vi "Auton Unbundle Array.vi"(10 "index (col)":i32, 11 "array":dbl[][](array[numeric])) -> (0 "Left Drive":dbl, 1 "Right Drive":dbl, 2 "Right Encoder":dbl, 3 "Auton Left Arm":dbl, 4 "Left Encoder":dbl, 5 "Auton Right Arm":dbl, 6 "Gripper":dbl)   [LabVIEW 2014]
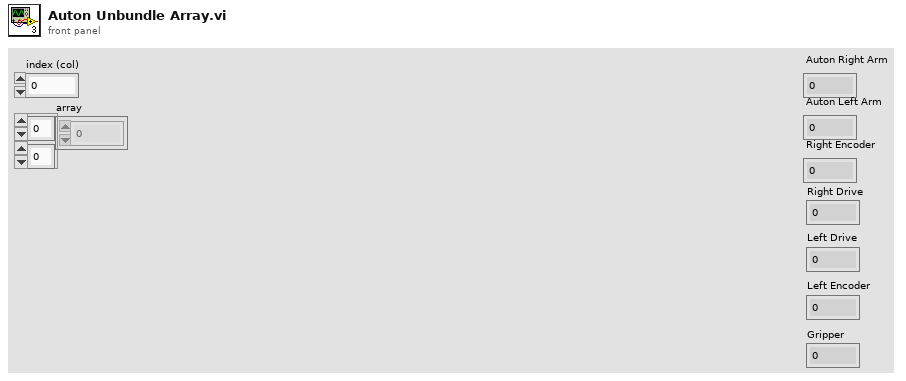
[diagram p1: front panel]
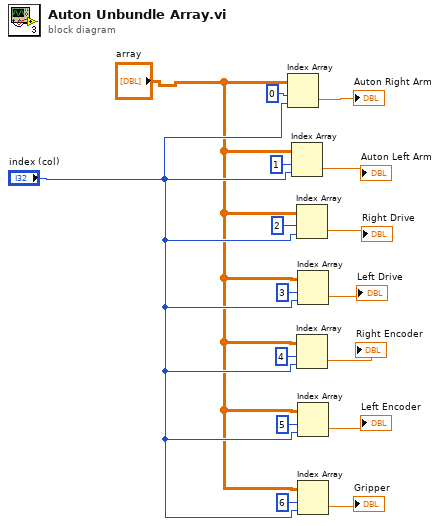
[diagram p0: block diagram]
diagram:
  n1 = Index Array(array="array", index (row)=0, index (col)="index (col)") -> (element=→"Auton Right Arm":dbl)
  n2 = Index Array(array="array", index (row)=1, index (col)="index (col)") -> (element=→"Auton Left Arm":dbl)
  n3 = Index Array(array="array", index (row)=2, index (col)="index (col)") -> (element=→"Right Drive":dbl)
  n4 = Index Array(array="array", index (row)=4 ("index"), index (col)="index (col)") -> (element=→"Right Encoder":dbl)
  n5 = Index Array(array="array", index (row)=3 ("index"), index (col)="index (col)") -> (element=→"Left Drive":dbl)
  n6 = Index Array(array="array", index (row)=5 ("index"), index (col)="index (col)") -> (element=→"Left Encoder":dbl)
  n7 = Index Array(array="array", index (row)=6 ("index"), index (col)="index (col)") -> (element=→"Gripper":dbl)
